vi "Process.vi"(8 "error in (no error)":errorcluster, 10 "Entry Console Start Msg in":refnum<class "Register Entry Console References.lvclass">, 11 "Architecture.lvlib:Thread.lvclass":refnum<class "Thread.lvclass">) -> (0 "error out":errorcluster, 1 "Stop?":bool, 3 "Architecture.lvlib:Thread.lvclass 2":refnum<class "Thread.lvclass">)   [LabVIEW 2013, in "Car Wash Controller.lvlib" / "Register Entry Console References.lvclass"]
uses:
  Register Entry Console References.lvclass
  Message.lvclass
  Thread.lvclass
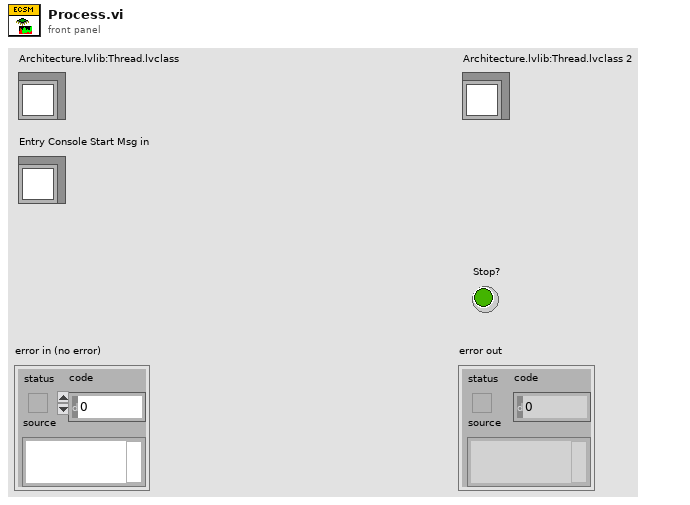
[diagram p1: front panel]
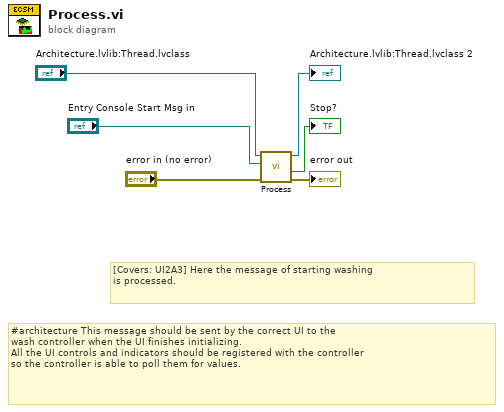
[diagram p0: block diagram]
diagram:
  # "#architecture This message should be sent by the correct UI to the \nwash controller when the UI finishes initializing.\nAll the UI controls and indicators should be registered with the controller\nso the controller is able to poll them for values."
  # "[Covers: UI2A3] Here the message of starting washing \nis processed."
  n1 = call-parent "Process.vi"("error in (no error)"="error in (no error)", "Message in"="Entry Console Start Msg in", "Architecture.lvlib:Thread.lvclass"="Architecture.lvlib:Thread.lvclass") -> ("error out"=→"error out":errorcluster, "Stop?"=→"Stop?":bool, "Architecture.lvlib:Thread.lvclass 2"=→"Architecture.lvlib:Thread.lvclass 2":refnum<class "Thread.lvclass">)  [unwired: 6 in]
